vi "Task Start.vi"(8 "error in (no error)":errorcluster, 11 "DebugGUI in":refnum<class "DebugGUI.lvclass">) -> (0 "error out":errorcluster, 3 "DebugGUI out":refnum<class "DebugGUI.lvclass">)   [LabVIEW 2020, in "Volatus.lvlib" / "DebugGUI.lvclass"]
uses:
  DebugGUI.lvclass
  DebugGUI.lvclass/DebugGUI.ctl
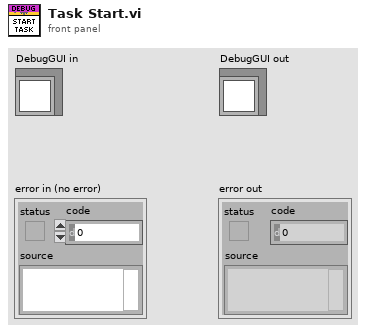
[diagram p1: front panel]
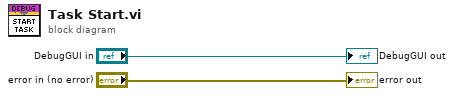
[diagram p0: block diagram]
diagram:
  "error out" <- "error in (no error)"
  "DebugGUI out" <- "DebugGUI in"
